vi "Simulation Input Global.vi"() -> ()   [LabVIEW 2014, in "Elevator System.lvlib"]
uses:
  Elevator System.lvlib
panel:
  in  "Sim Gripper Input R":dbl
  in  "Sim Gripper Input L":dbl
  in  "Sim Elevator Input":dbl
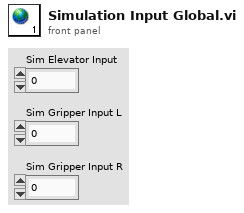
[diagram p1: front panel]
diagram:
